vi "I-SRC Configure.vi"(5 "Voltage Limit":dbl, 7 "Current Level":dbl, 8 "error in (no error)":errorcluster, 11 "VISA resource name in":refnum<visa-resource-name>) -> (0 "error out":errorcluster, 3 "VISA resource name out":refnum<visa-resource-name>)   [LabVIEW 2016, in "Hall Effect Library.lvlib"]
uses:
  Hall Effect Library.lvlib
  Global Variables/Instruments.vi
  I-SRC Configure (622X).vi
  I-SRC Configure (26XX).vi
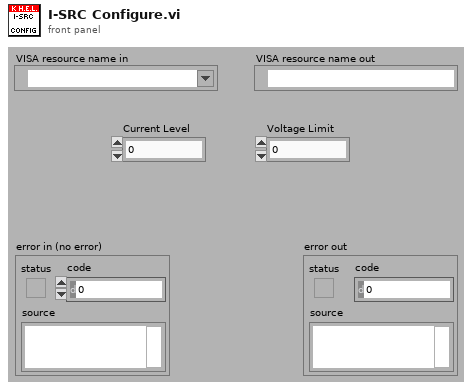
[diagram p1: front panel]
types:
  T1 = typedef "Hall Effect Library.lvlib/I-Sources.ctl" = enum16{"622X", "26XX"}
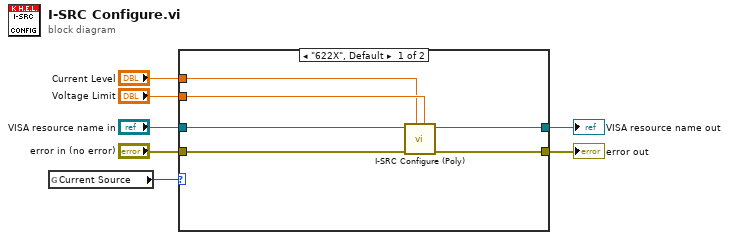
[diagram p0: block diagram]
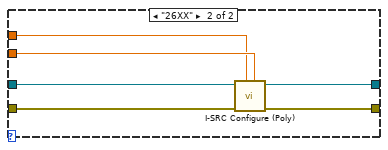
[diagram p2: hidden frame]
diagram:
  n1 = global read "Instruments.vi" "Current Source"() -> (w7:T1)
  n2 = case shown="\"622X\", Default" w7 {
    tunnel: "VISA resource name in" -> [w13 w19]
    tunnel: [w12 w18] -> w5
    tunnel: [w11 w17] -> w4
    tunnel: "error in (no error)" -> [w10 w16]
    tunnel: "Voltage Limit" -> [w9 w15]
    tunnel: "Current Level" -> [w8 w14]
    frame "622X", Default {
      n3 = call-poly "I-SRC Configure (Poly).vi"("Voltage Limit"=w9, "Current Level"=w8, "error in (no error)"=w10, "VISA resource name in"=w13) -> ("error out"=w11:errorcluster, "VISA resource name out"=w12:refnum<visa-resource-name>)  [unwired: 6 out]
    }
    frame "26XX" {
      n4 = call-poly "I-SRC Configure (Poly).vi"("Voltage Limit"=w15, "Current Level"=w14, "error in (no error)"=w16, "VISA resource name in"=w19) -> ("error out"=w17:errorcluster, "VISA resource name out"=w18:refnum<visa-resource-name>)  [unwired: 6 out]
    }
  }
  "error out" <- w4
  "VISA resource name out" <- w5
